vi "merge_SR Bistable.vi"   [LabVIEW 2017, in "NI_FunctionBlockMergeVIs.lvlib"]
doc: "Creates a set-dominant latch, also known as a flip-flop."
uses:
  <vilib>/functionblocks/NI_FunctionBlockMergeVIs.lvlib
  <vilib>/functionblocks/FB Core/FB Core.xnode
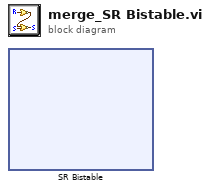
[diagram p0: block diagram]
diagram:
  n1 = xnode "SR Bistable"() -> ()  [unwired: 3 in, 2 out]
